vi "Edit Layer.vi"(8 "error in (no error)":errorcluster, 9 "Layer Index":i16, 10 "ShapeRef":refnum<data-value>, 11 "Image in":refnum<class "Image.lvclass">) -> (0 "error out":errorcluster, 3 "Image out":refnum<class "Image.lvclass">)   [LabVIEW 2017, in "LV Image Editor Framework.lvlib" / "Image.lvclass"]
uses:
  <vilib>/LIEF/Image/Image.lvclass
  <vilib>/LIEF/Forms/Shape/Shape.lvclass
  <vilib>/LIEF/Image/Image.lvclass/Image.ctl
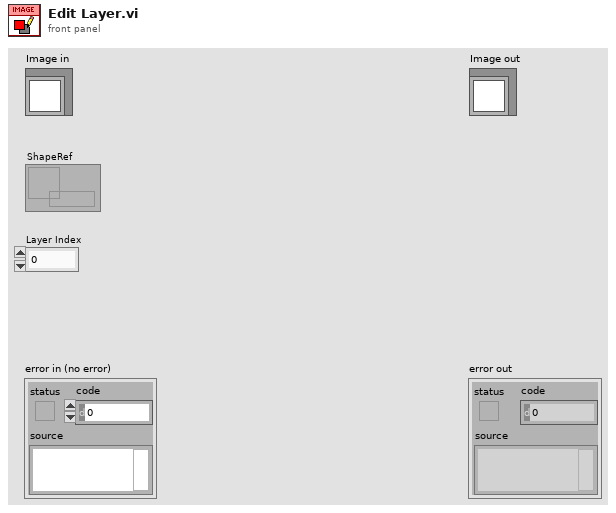
[diagram p1: front panel]
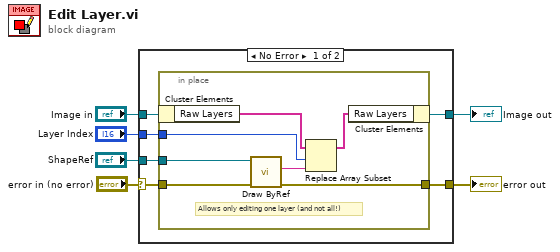
[diagram p0: block diagram]
diagram:
  n1 = case shown="No Error" "error in (no error)" {
    selector: "error in (no error)" -> [w8 w21]
    tunnel: [w7 w21] -> w5
    tunnel: [w10 w20] -> w3
    tunnel: "Image in" -> [w12 w20]
    tunnel: "Layer Index" -> [w11 _]
    tunnel: "ShapeRef" -> [w9 _]
    frame No Error {
      n2 = in-place {
        in-place-border: w11 -> [w15]
        in-place-border: w9 -> [w17]
        in-place-border: w8 -> [w14]
        in-place-border: [w13] -> w7
        # "Allows only editing one layer (and not all!)"
        n3 = in-place-cluster #1(w12) -> ("Raw Layers"=w19:string[])
        n4 = call <vilib>:"Draw ByRef.vi"("error in (no error)"=w14, "ShapeRef"=w17) -> ("error out"=w13:errorcluster, "Raw Image"=w16:string)  [unwired: 7 in, 1 out]
        n5 = Replace Array Subset(array=w19, new element=w16, index=w15) -> (w18:string[])
        n6 = in-place-cluster #1("Raw Layers"=w18) -> (w10:refnum<class "Image.lvclass">)
      }
    }
    frame Error {
    }
  }
  "error out" <- w5
  "Image out" <- w3
